vi "AutoToggle.vi"(8 "error in":T1) -> ()   [LabVIEW 2014]
uses:
  ErrorOut.ctl
  Robot Global Data.vi
  <vilib>/Rock Robotics/Network Tables/SD Write Boolean.vi
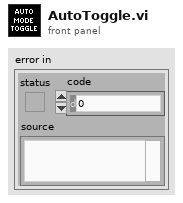
[diagram p1: front panel]
types:
  T1 = typedef "ErrorOut.ctl" = errorcluster
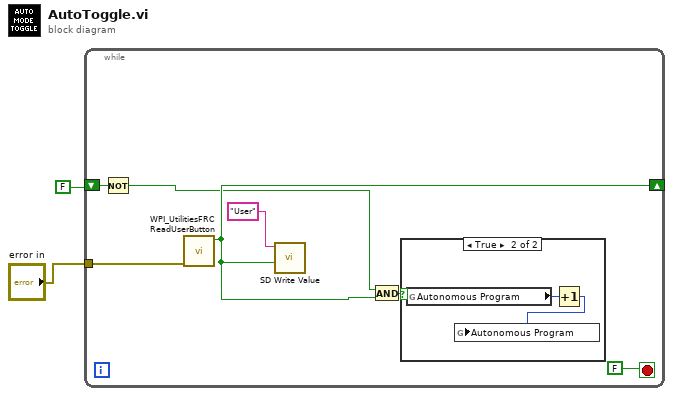
[diagram p0: block diagram]
diagram:
  n1 = while {
    tunnel: "error in" -> [w8]
    shift-right: [w4] -> _
    shift-left: FALSE -> [w6]
    stop <- FALSE stop-if-true
    n2 = Not(x=w6) -> (.not. x?=w3:bool)
    n3 = call <vilib>:"WPI_UtilitiesFRC ReadUserButton.vi"("error in"=w8) -> ("User Button"=w4:bool)  [unwired: 9 in, 1 out]
    n4 = call-poly <vilib>:"SD Write Value.vi"("Boolean"=w4, "Name"="User") -> ()  [unwired: 8 in, 2 out]
    n5 = And(x=w3, y=w4) -> (x .and. y?=w5:bool)
    n6 = case shown="True" w5 {
      frame False {
      }
      frame True {
        n7 = global read "Robot Global Data.vi" "Autonomous Program"() -> (w11:enum16{"Forward\n", "Stack", "Null"})
        n8 = Increment(x=w11) -> (x+1=w10:enum16{"Forward\n", "Stack", "Null"})
        n9 = global write "Robot Global Data.vi" "Autonomous Program"(w10) -> ()
      }
    }
  }
